vi "Waveform_Extract from StartEnd and Duration.vi"(8 "Error":errorcluster, 9 "Duration(S)":dbl, 10 "From End(f)\nFrom Beginning(t)":bool, 11 "Buffer":T2) -> (0 "Error Out":errorcluster, 1 "End Index Out":i32, 2 "Start Index Out":i32, 3 "Waveform Out":T1)   [LabVIEW 2016]
doc: "Retrieves a subset of a waveform at a specified time or index. You must manually select the polymorphic instance you want to use."
uses:
  TypeDefs_Utility/Ref_DVR_Buffer.ctl
  Universal Controls/Waveform_Data.ctl
  Universal Controls/Read Write Button.ctl
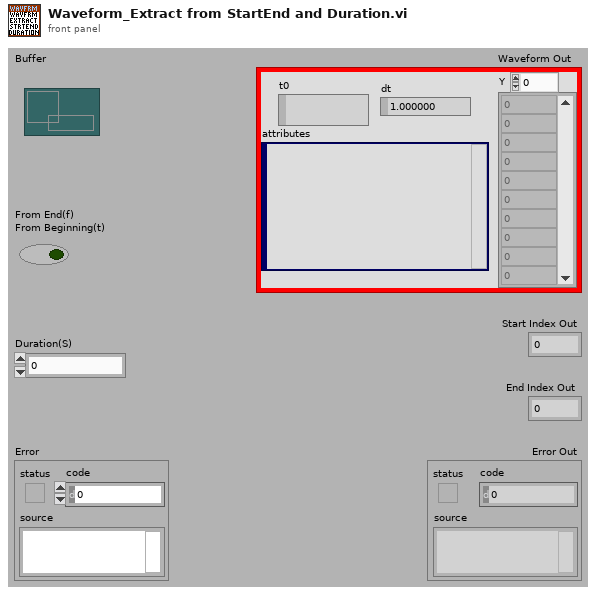
[diagram p1: front panel]
types:
  T1 = typedef "Waveform_Data.ctl" = waveform(dbl)
  T2 = typedef "Ref_DVR_Buffer.ctl" = refnum<data-value>
  T3 = typedef "Read Write Button.ctl" = bool
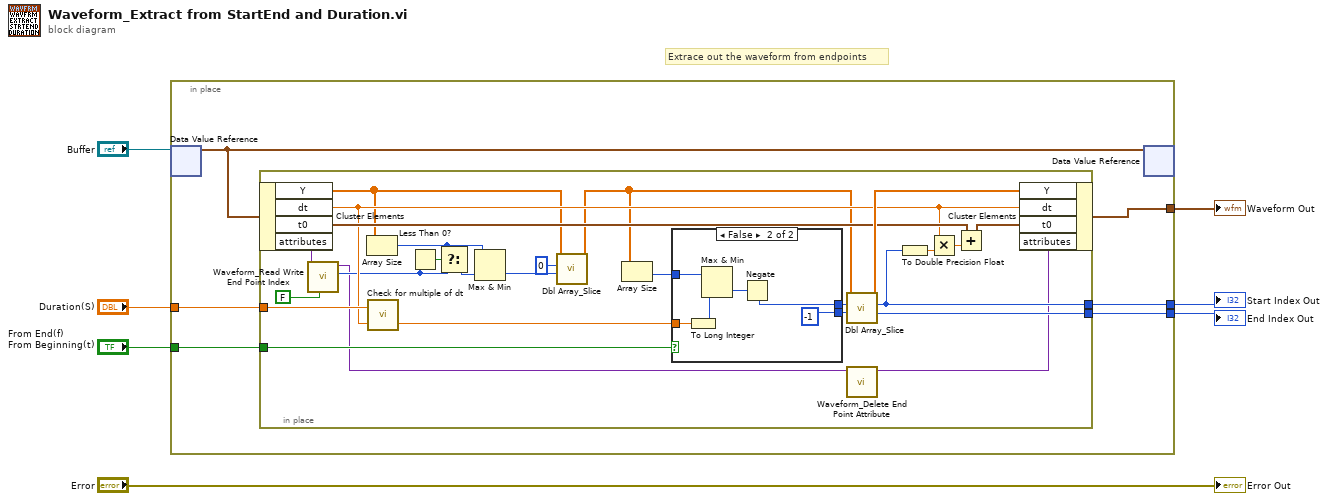
[diagram p0: block diagram]
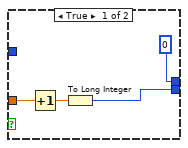
[diagram p2: hidden frame]
diagram:
  # "Extrace out the waveform from endpoints"
  n1 = in-place {
    in-place-border: [w13] -> w6
    in-place-border: [w12] -> w5
    in-place-border: [w11] -> w4
    in-place-border: "From End(f)\nFrom Beginning(t)" -> [w10]
    in-place-border: "Duration(S)" -> [w9]
    n2 = in-place-dvr #1("Buffer") -> (w8:T1)  [unwired: 1 out]
    n3 = in-place {
      in-place-border: [w27] -> w12
      in-place-border: [w35] -> w11
      in-place-border: w10 -> [w34]
      in-place-border: w9 -> [w33]
      n4 = in-place-cluster #2(w8) -> ("Y"=w23:dbl[], "dt"=w32:dbl, "t0"=w37:timestamp, "attributes"=w15:variant)
      n5 = call "Waveform_Read Write End Point Index.vi"("Read(f)\nWrite(t)"=T3 FALSE ("Read(f)\nWrite(t)"), "Waveform Atributes"=w15) -> ("End Point Out"=w17:i32, "Waveform Atributes Out"=w14:variant)  [unwired: 7 in, 1 out]
      n6 = Array Size(array=w23) -> (size(s)=w24:i32)
      n7 = call <vilib>:"Check for multiple of dt.vi"("dt"=w32, "time"=w33) -> ("iQuotient"=w31:dbl)  [unwired: 1 out]
      n8 = Less Than 0?(x=w17) -> (x < 0?=w26:bool)
      n9 = Select(t=w24, s=w26, f=w17) -> (s? t:f=w25:i32)
      n10 = Max & Min(x=w24, y=w25) -> (min(x,y)=w22:i32)  [unwired: 1 out]
      n11 = call "Dbl Array_Slice.vi"("End Index\n(-1) Last point"=w22, "Start Index"=0, "Array"=w23) -> ("Subarray (array[i:j]) Out"=w19:dbl[])  [unwired: 1 in, 7 out]
      n12 = Array Size(array=w19) -> (size(s)=w20:i32)
      n13 = case shown="False" w34 {
        tunnel: [0 ("Start") w47] -> w29
        tunnel: w31 -> [w42 w48]
        tunnel: [w40 -1 ("Start")] -> w30
        tunnel: w20 -> [_ w44]
        frame True {
          n14 = Increment(x=w42) -> (x+1=w41:dbl)
          n15 = To Long Integer(number=w41) -> (32bit integer=w40:i32)
        }
        frame False {
          n16 = To Long Integer(number=w48) -> (32bit integer=w46:i32)
          n17 = Max & Min(x=w44, y=w46) -> (min(x,y)=w45:i32)  [unwired: 1 out]
          n18 = Negate(x=w45) -> (-x=w47:i32)
        }
      }
      n19 = call "Dbl Array_Slice.vi"("End Index\n(-1) Last point"=w30, "Start Index"=w29, "Array"=w19) -> ("End Out"=w35:i32, "Start Out"=w27:i32, "Subarray (array[i:j]) Out"=w39:dbl[])  [unwired: 1 in, 5 out]
      n20 = call "Waveform_Delete End Point Attribute.vi"("Waveform Atributes"=w14) -> ("Waveform Atributes Out"=w16:variant)  [unwired: 9 in, 1 out]
      n21 = To Double Precision Float(number=w27) -> (double precision float=w28:dbl)
      n22 = Multiply(x=w32, y=w28) -> (x*y=w38:dbl)
      n23 = Add(x=w37, y=w38) -> (x+y=w36:timestamp)
      n24 = in-place-cluster #2("Y"=w39, "dt"=w32, "t0"=w36, "attributes"=w16) -> (w13:T1)
    }
    n25 = in-place-dvr #1(w8) -> ()  [unwired: 2 out]
  }
  "Waveform Out" <- w6
  "Start Index Out" <- w5
  "End Index Out" <- w4
  "Error Out" <- "Error"
